vi "getOdoDirection.vi"(8 "error in (no error)":errorcluster, 11 "pHandle":u32) -> (0 "error out":errorcluster, 1 "return type":i32, 3 "odoDirectionStr":string)   [LabVIEW 2011, in "sbgLabView.lvlib"]
uses:
  sbgLabView.lvlib
  sbgMatLab.dll
panel:
  in  "channel":u8
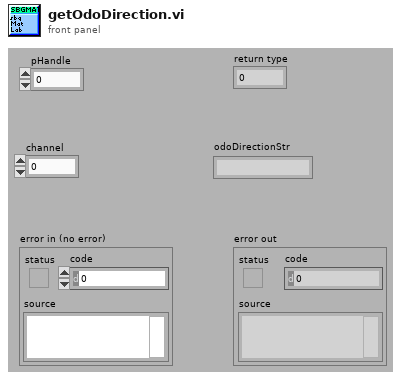
[diagram p1: front panel]
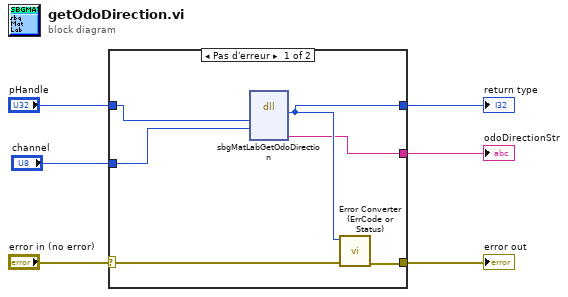
[diagram p0: block diagram]
diagram:
  n1 = case shown="Pas d'erreur" "error in (no error)" {
    selector: "error in (no error)" -> [w9 w13]
    tunnel: [w8 w13] -> w5
    tunnel: [w12 _] -> w4
    tunnel: "pHandle" -> [w11 _]
    tunnel: [w10 _] -> w2
    tunnel: "channel" -> [w7 _]
    frame No Error {
      n2 = dll-call lib="C:/SBG-Systems/remote/projects/software/projects/labviewExample/sbgLabView/sbgMatLab.*" fn="sbgMatLabGetOdoDirection" ("sbgMatLab.dll:sbgMatLabGetGpsOptions")("pHandle"=w11, "channel"=w7) -> ("type de retour"=w12:i32, "odoDirectionStr"=w10:string)  [unwired: 6 in, 2 out]
      n3 = call "Error Converter (ErrCode or Status).vi"("error in (no error)"=w9, "error code"=w12) -> ("error out"=w8:errorcluster)  [unwired: 9 in]
    }
    frame Error {
    }
  }
  "return type" <- w4
  "odoDirectionStr" <- w2
  "error out" <- w5
